vi "Serial.Parse PNPDeviceID.vi"(11 "String":string) -> (1 "PID":string, 2 "VID":string, 3 "Type":string)   [LabVIEW 2018]
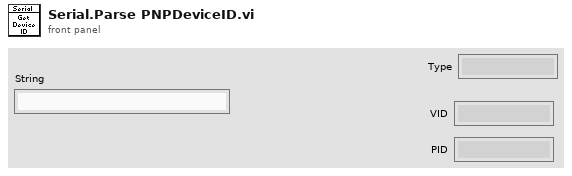
[diagram p1: front panel]
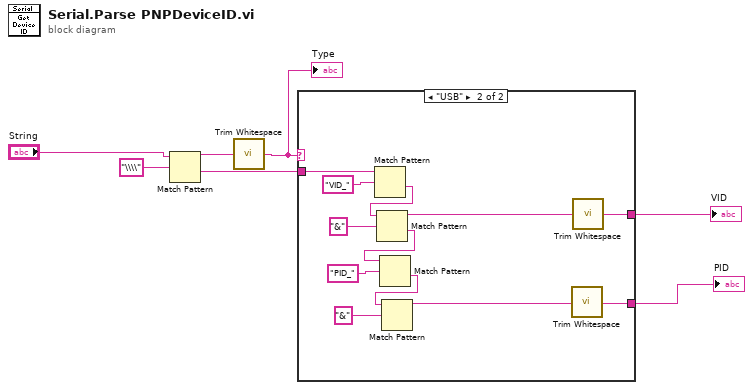
[diagram p0: block diagram]
diagram:
  n1 = Match Pattern(string="String", regular expression="\\\\") -> (before substring=w6:string, after substring=w3:string)  [unwired: 1 in, 2 out]
  n2 = call <vilib>:"Trim Whitespace.vi"("string"=w6) -> ("trimmed string"=w4:string)  [unwired: 1 in]
  "Type" <- w4
  n3 = case shown="\"USB\"" w4 {
    tunnel: w3 -> [_ w19]
    tunnel: [_ w10] -> w2
    tunnel: [_ w11] -> w1
    frame "False", Default {
    }
    frame "USB" {
      n4 = Match Pattern(string=w19, regular expression="VID_") -> (after substring=w16:string)  [unwired: 1 in, 3 out]
      n5 = Match Pattern(string=w16, regular expression="&") -> (before substring=w9:string, after substring=w12:string)  [unwired: 1 in, 2 out]
      n6 = Match Pattern(string=w12, regular expression="PID_") -> (after substring=w15:string)  [unwired: 1 in, 3 out]
      n7 = Match Pattern(string=w15, regular expression="&") -> (before substring=w8:string)  [unwired: 1 in, 3 out]
      n8 = call <vilib>:"Trim Whitespace.vi"("string"=w8) -> ("trimmed string"=w11:string)  [unwired: 1 in]
      n9 = call <vilib>:"Trim Whitespace.vi"("string"=w9) -> ("trimmed string"=w10:string)  [unwired: 1 in]
    }
  }
  "VID" <- w2
  "PID" <- w1
